vi "adam-DO-send-command.vi"(6 "Stop All":bool, 7 "Device Address":dbl=1.0, 8 "error in (no error)":errorcluster, 9 "Channel Active":bool, 10 "Channel Number":dbl=1.0, 11 "VISA Refnum in":refnum<visa-resource-name>) -> (0 "error out":errorcluster, 1 "Desired State":bool, 2 "command":string, 3 "VISA Refnum out":refnum<visa-resource-name>, 4 "STOPPED":bool, 5 "Bytes Written":u32)   [LabVIEW 2024]
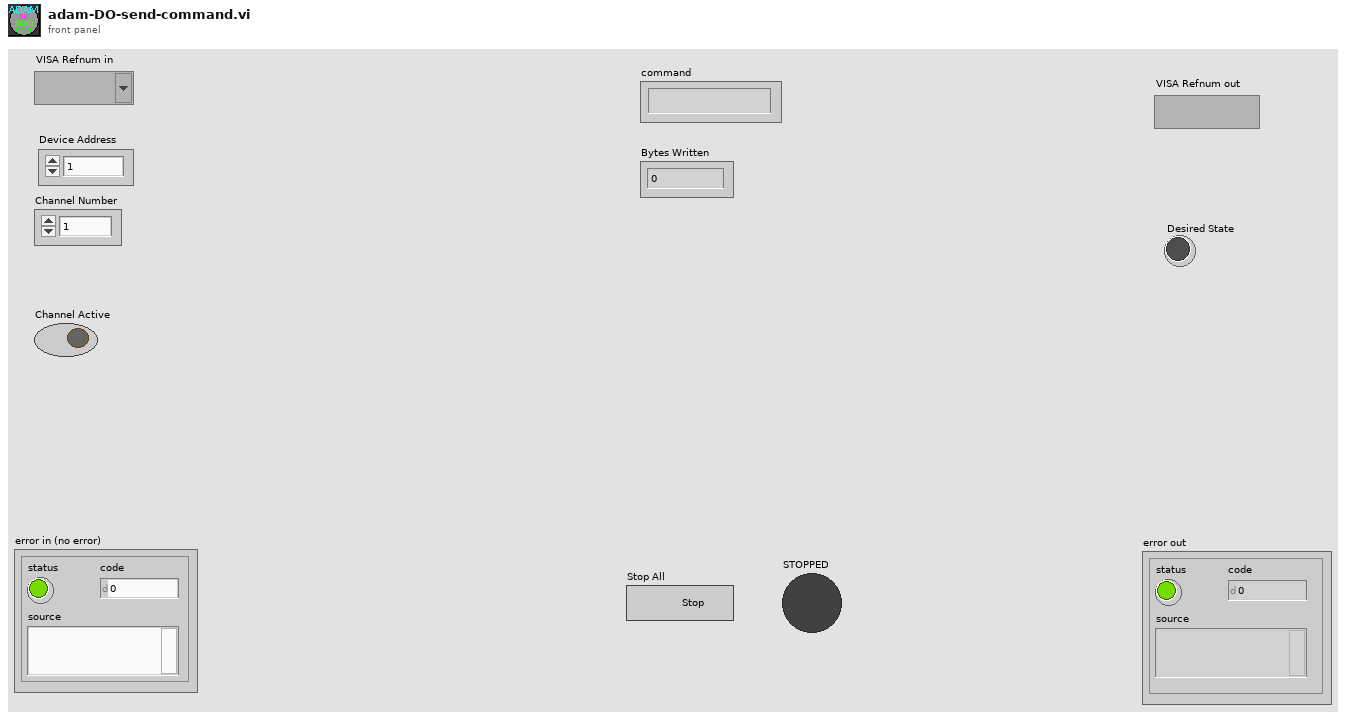
[diagram p1: front panel]
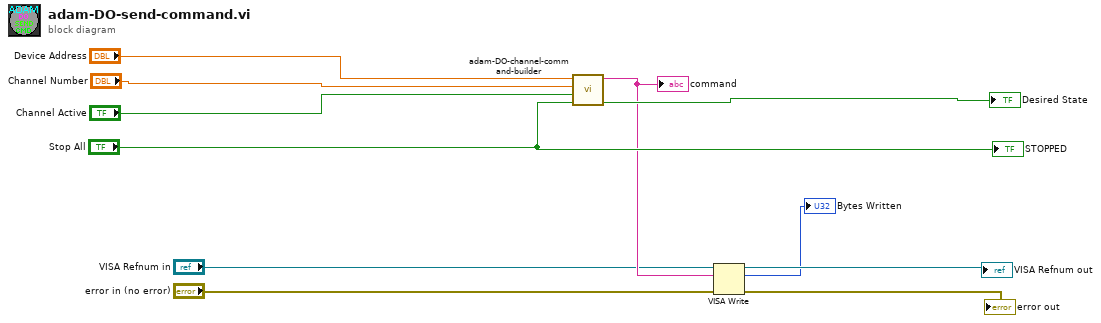
[diagram p0: block diagram]
diagram:
  n1 = call "adam-DO-channel-command-builder.vi"("Stop All"="Stop All", "Channel Active"="Channel Active", "Channel Number"="Channel Number", "Device Address"="Device Address") -> ("Desired State"=→"Desired State":bool, "concatenated command"=w9:string)  [unwired: 6 in]
  "command" <- w9
  n2 = VISA Write(VISA resource name="VISA Refnum in", write buffer=w9, error in (no error)="error in (no error)") -> (VISA resource name out=→"VISA Refnum out":refnum<visa-resource-name>, return count=→"Bytes Written":u32, error out=→"error out":errorcluster)
  "STOPPED" <- "Stop All"
